vi "DCA Build Query - DataFinder.vi"(8 "error in (no error)":errorcluster, 10 "UserName":string, 11 "Fields":T2[](array[typedef])) -> (0 "error out":errorcluster, 3 "Field Information":T1[](array[typedef]))   [LabVIEW 2011]
uses:
  server/DIAdem/lib/DIAdem Query Data.ctl
  server/DataFinder/DataFinder Comparisons.ctl
  cgi-bin/_cgi-lib/TDM_INDEX Record.ctl
  server/DataFinder/eSearch Types.ctl
  server/DataFinder/Datafinder Query.ctl
  server/DIAdem/Datasheet/Query Parameters.ctl
  server/DIAdem/lib/DIAdem Query Queue.ctl
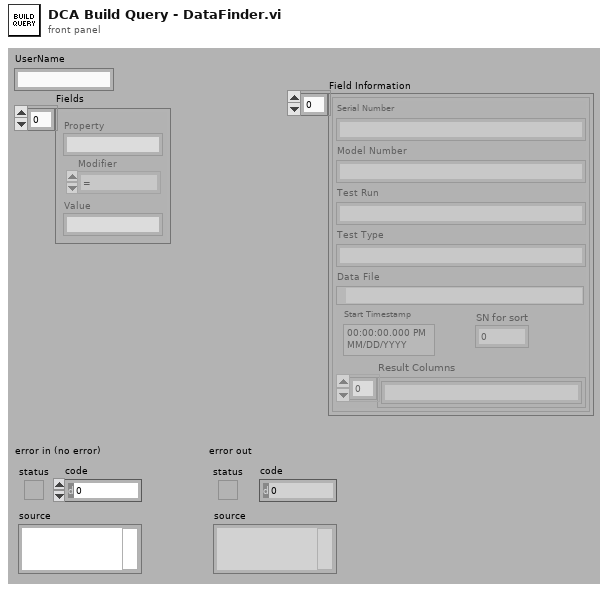
[diagram p1: front panel]
types:
  T1 = typedef "TDM_INDEX Record.ctl" = cluster{"Model Number":string, "SN for sort":i32, "Test Type":string, "Test Run":string, "Serial Number":string, "Start Timestamp":timestamp, "Data File":path, "Result Columns":string[]}
  T2 = typedef "DIAdem Query Data.ctl" = cluster{"Property":string, "Modifier":T3, "Value":string}
  T3 = typedef "DataFinder Comparisons.ctl" = enum16{"=", "<>", "<", "<=", ">", ">="}
  T4 = typedef "DIAdem Query Queue.ctl" = cluster{"UserName":string, "Search Parameters":T5[], "eSearch Type":T6, "Query Name (vbs)":string, "Response queue name":string, "Logic String":string}
  T5 = typedef "Datafinder Query.ctl" = cluster{"eSearch Types":T6, "Property Name":string, "DataFinder Comparisons":T3, "Property Value":string}
  T6 = typedef "eSearch Types.ctl" = enum16{"eSearchFile", "eSearchChannelGroup", "eSearchChannel"}
  T7 = typedef "Query Parameters.ctl" = cluster{"Action":string, "Serial Number":string, "Model Number":string, "MNWILD":string, "StartDate":string, "EndDate":string, "DateCOMP":string, "Conditions":T5[], "MN Wild List":string[], "SN by MN Wild List":cluster{"Serial Number List":string[]}[], "Recall Table?":bool, "Type":string, "Show Date?":bool, "Show Conditions?":bool, "Serial Number Display Name":string, "Model Number Display Name":string, "Test Type String":string, "Manager":bool, "Custom Rows":string[][], "Custom Result HTML":string, "User Name":string, "State":string, "MN Query ":string, "SN Query":string, "Custom Analysis HTML":string, "RUNSELECT":string}
  T8 = typedef "Connection Refnum.ctl" = cluster{"Environment Handle":i32, "Connection Handle":i32}
  T9 = typedef "DIAdem Query Result.ctl" = cluster{"Results":string[][], "# of Items":i32, "Data Returned?":bool, "Result TDM":path, "Timed Out?":bool}
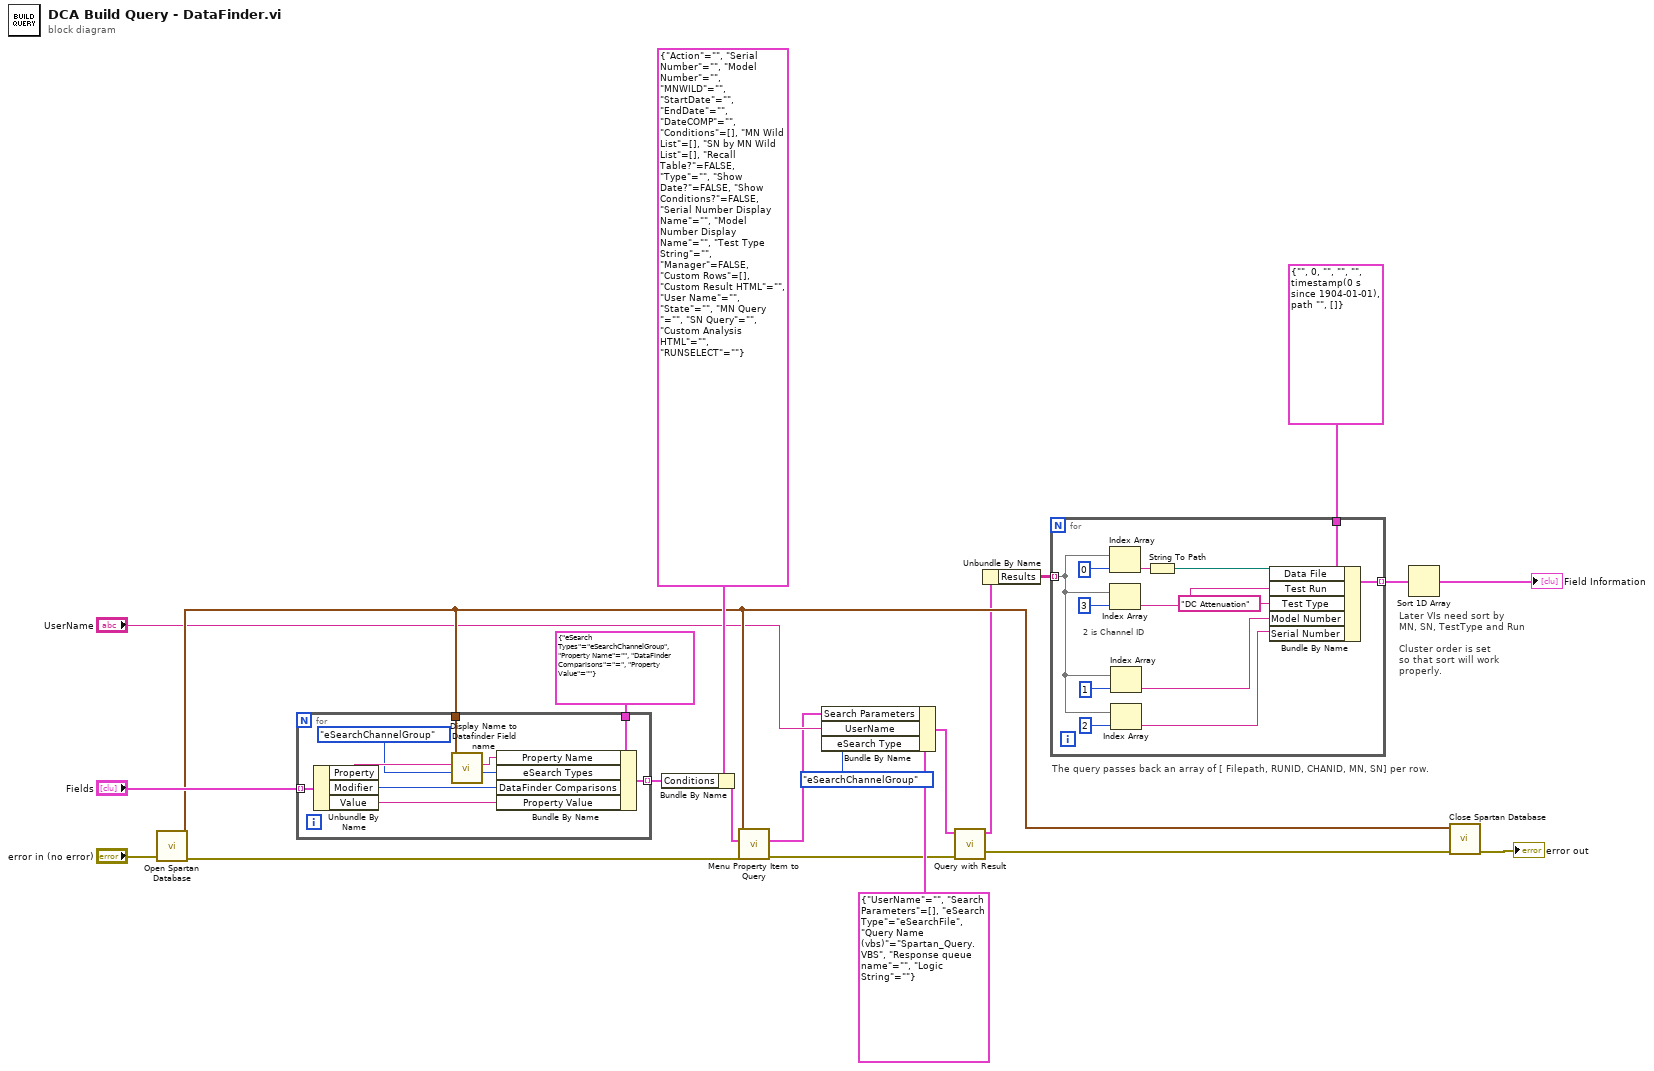
[diagram p0: block diagram]
diagram:
  # "The query passes back an array of [ Filepath, RUNID, CHANID, MN, SN] per row."
  # "Later VIs need sort by \nMN, SN, TestType and Run\n\nCluster order is set\nso that sort will work\nproperly."
  n1 = call "Open Spartan Database.vi"("error in (no error)"="error in (no error)") -> ("error out"=w12:errorcluster, "Connection Refnum"=w10:T8)  [unwired: 1 in, 8 out]
  n2 = for {
    tunnel: "Fields" -> [w31] mode=indexing
    tunnel: [w28] -> w15 mode=indexing
    tunnel: T5 {"eSearch Types"=enum."eSearchChannelGroup", "Property Name"="", "DataFinder Comparisons"=enum."=", "Property Value"=""} ("Data Finder Parameters") -> [w27]
    tunnel: w10 -> [w22]
    n3 = Unbundle By Name(w31) -> ("Property"=w26:string, "Modifier"=w30:T3, "Value"=w29:string)
    n4 = call "Display Name to Datafinder Field name.vi"("eSearch Type In"=eSearch_Types."eSearchChannelGroup" ("eSearch Types"), "Field Display Name"=w26, "Connection Refnum"=w22) -> ("eSearch Type Out"=w23:T6, "Datafinder Search Name"=w24:string)  [unwired: 1 in, 6 out]
    n5 = Bundle By Name(cluster=w27, "Property Name"=w24, "eSearch Types"=w23, "DataFinder Comparisons"=w30, "Property Value"=w29) -> (w28:T5)
  }
  n6 = Bundle By Name(cluster=T7 {"Action"="", "Serial Number"="", "Model Number"="", "MNWILD"="", "StartDate"="", "EndDate"="", "DateCOMP"="", "Conditions"=[], "MN Wild List"=[], "SN by MN Wild List"=[], "Recall Table?"=FALSE, "Type"="", "Show Date?"=FALSE, "Show Conditions?"=FALSE, "Serial Number Display Name"="", "Model Number Display Name"="", "Test Type String"="", "Manager"=FALSE, "Custom Rows"=[], "Custom Result HTML"="", "User Name"="", "State"="", "MN Query "="", "SN Query"="", "Custom Analysis HTML"="", "RUNSELECT"=""} ("Custom Search Parameters"), "Conditions"=w15) -> (w14:T7)
  n7 = call "Menu Property Item to Query.vi"("error in (no error)"=w12, "Custom Search Parameters"=w14, "Connection Refnum In"=w10) -> ("error out"=w3:errorcluster, "Custom Search Parameters"=w1:T5[])  [unwired: 7 out]
  n8 = Bundle By Name(cluster=T4 {"UserName"="", "Search Parameters"=[], "eSearch Type"=enum."eSearchFile", "Query Name (vbs)"="Spartan_Query.VBS", "Response queue name"="", "Logic String"=""} ("Query Parameter Data"), "Search Parameters"=w1, "UserName"="UserName", "eSearch Type"=eSearch_Types."eSearchChannelGroup" ("eSearch Types")) -> (w8:T4)
  n9 = call "Query with Result.vi"("error in (no error)"=w3, "Query Parameter Data"=w8) -> ("error out"=w2:errorcluster, "Query Return Data"=w5:T9)  [unwired: 8 out]
  n10 = Unbundle By Name(w5) -> ("Results"=w4:string[][])
  n11 = for {
    tunnel: w4 -> [w36] mode=indexing
    tunnel: T1 {"Model Number"="", "SN for sort"=0, "Test Type"="", "Test Run"="", "Serial Number"="", "Start Timestamp"=timestamp(0 s since 1904-01-01), "Data File"=path "", "Result Columns"=[]} ("Station Information") -> [w44]
    tunnel: [w39] -> w19 mode=indexing
    # "2 is Channel ID"
    n12 = Index Array(array=w36, index=0) -> (element=w41:string)
    n13 = Index Array(array=w36, index=3) -> (element=w40:string)
    n14 = Index Array(array=w36, index=1) -> (element=w35:string)
    n15 = Index Array(array=w36, index=2) -> (element=w34:string)
    n16 = String To Path(string=w41) -> (path=w33:path)
    n17 = Bundle By Name(cluster=w44, "Data File"=w33, "Test Run"=w40, "Test Type"="DC Attenuation", "Model Number"=w35, "Serial Number"=w34) -> (w39:T1)
  }
  n18 = Sort 1D Array(array=w19) -> (sorted array=→"Field Information":T1[])
  n19 = call "Close Spartan Database.vi"("error in (no error)"=w2, "Connection Refnum"=w10) -> ("error out"=→"error out":errorcluster)  [unwired: 2 in, 7 out]
